vi "MOTION_ARDUNIO_LABVIEW_RXTX.vi"() -> ()   [LabVIEW 2014]
uses:
  <vilib>/Instr/_visa.llb/VISA Configure Serial Port (Instr).vi
panel:
  in  "stop bits (10: 1 bit)":u16(ring)=10 items=["1.0"=10, "1.5"=15, "2.0"=20]
  in  "parity (0:none)":enum16{"None", "Odd", "Even", "Mark", "Space"}(ring)
  in  "data bits (8)":u16=8 min=5 max=8 step=1
  in  "baud rate (9600)":u32=9600
  out "?":bool
  out "?":bool
  out "NO MOTION DETECTED":bool
  out "MOTION DETECTED":bool
  in  "stop":bool
  out "Waveform Chart":i32(graph)
  out "MOTION LEVEL VARIABLE":string
  out "read buffer":string
  in  "byte count":u32
  in  "VISA resource name":refnum<visa-resource-name>
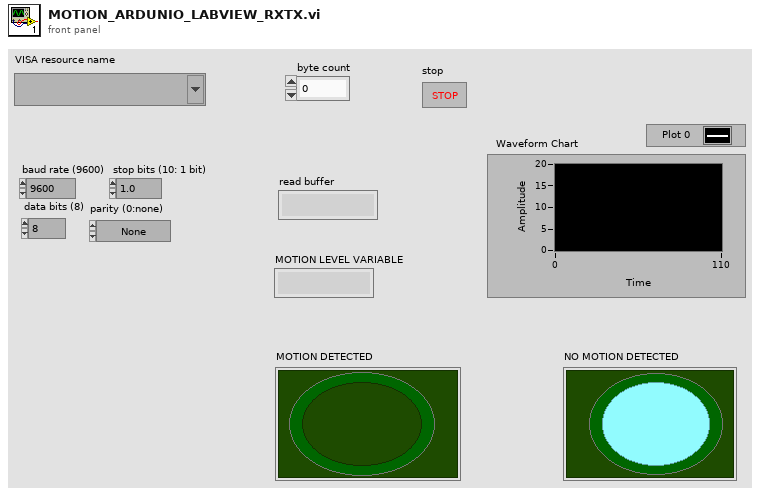
[diagram p1: front panel]
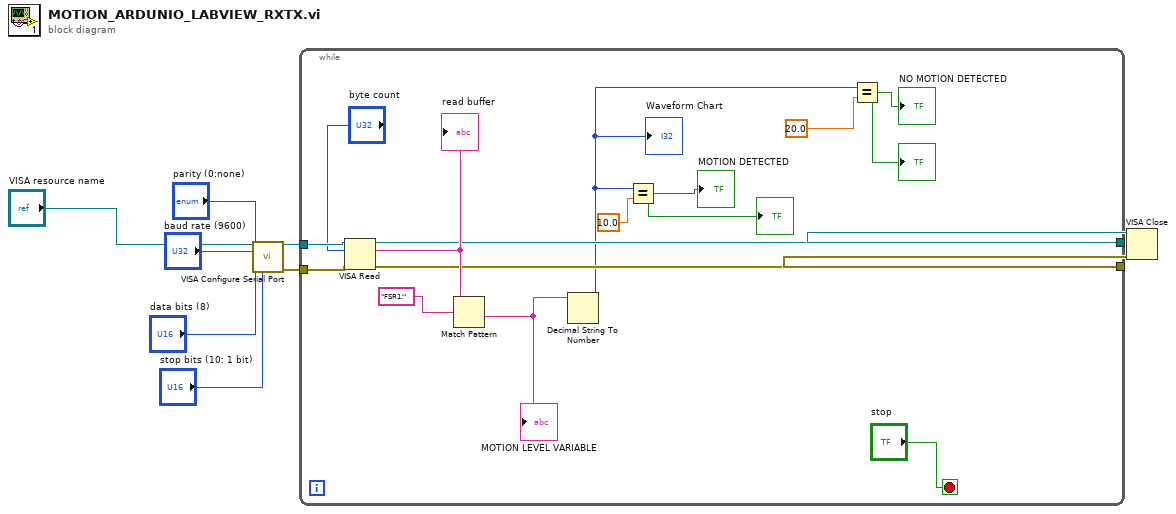
[diagram p0: block diagram]
diagram:
  n1 = call-poly "VISA Configure Serial Port"("VISA resource name"="VISA resource name", "baud rate (9600)"="baud rate (9600)", "data bits (8)"="data bits (8)", "parity (0:none)"="parity (0:none)", "stop bits (10: 1 bit)"="stop bits (10: 1 bit)") -> ("VISA resource name out"=w8:refnum<visa-resource-name>, "error out"=w7:errorcluster)  [unwired: 9 in]
  n2 = while {
    tunnel: w8 -> [w23]
    tunnel: w7 -> [w22]
    tunnel: [w18] -> w6
    tunnel: [w17] -> w5
    stop <- "stop" stop-if-true
    n3 = VISA Read(VISA resource name=w23, byte count="byte count", error in (no error)=w22) -> (VISA resource name out=w17:refnum<visa-resource-name>, read buffer=w20:string, error out=w18:errorcluster)  [unwired: 1 out]
    "read buffer" <- w20
    n4 = Match Pattern(string=w20, regular expression="FSR1:") -> (after substring=w13:string)  [unwired: 1 in, 3 out]
    "MOTION LEVEL VARIABLE" <- w13
    n5 = Decimal String To Number(string=w13) -> (number=w12:i32)  [unwired: 2 in, 1 out]
    "Waveform Chart" <- w12
    n6 = Equal?(x=w12, y=10.0) -> (x = y?=→"MOTION DETECTED" →"?":bool)
    n7 = Equal?(x=w12, y=20.0) -> (x = y?=→"NO MOTION DETECTED" →"?":bool)
  }
  n8 = VISA Close(VISA resource name=w5, error in (no error)=w6) -> ()  [unwired: 1 out]
